vi "Set Channel (Blue).vi"(8 "error in (no error)":errorcluster, 10 "Channel Data in":T1, 11 "ARGB Image in":T2) -> (0 "error out":errorcluster, 3 "ARGB Image":T2)   [LabVIEW 2020, in "image.lvlib"]
doc: "Set the channel of an ARGB Image"
uses:
  image.lvlib
  ARGB Image.ctl
  Greyscale Image.ctl
  ARGBChannels.ctl
  <vilib>/Utility/error.llb/Error Cluster From Error Code.vi
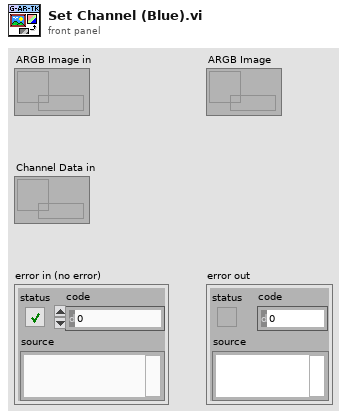
[diagram p1: front panel]
types:
  T1 = typedef "image.lvlib/Greyscale Image.ctl" = refnum<data-value>
  T2 = typedef "image.lvlib/ARGB Image.ctl" = refnum<data-value>
  T3 = typedef "image.lvlib/ARGBChannels.ctl" = enum8{"Blue", "Green", "Red", "Alpha"}
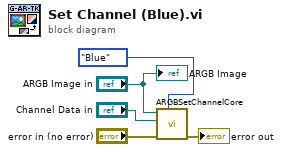
[diagram p0: block diagram]
diagram:
  n1 = call "ARGBSetChannelCore.vi"("Channels"=ARGBChannels."Blue" ("Extract_Operation"), "error in (no error)"="error in (no error)", "Channel Data in"="Channel Data in", "Image in"="ARGB Image in") -> ("error out"=→"error out":errorcluster)  [unwired: 7 in]
  "ARGB Image" <- "ARGB Image in"
